vi "Two_tanks.vi"() -> ()   [LabVIEW 2016]
uses:
  <vilib>/Simulation/Scripting/Companion Diagram/SimConfigNode/SimParams.ctl
  <vilib>/Simulation/Scripting/Companion Diagram/SimConfigNode/_simSolvers.ctl
  <vilib>/Simulation/Implementation/Shared/SIMSCR Execution Mode.ctl
  <vilib>/Simulation/Param Hierarchy/Typedefs/SIMPH Param Control Actions.ctl
  <vilib>/Simulation/Implementation/Shared/SIM limit type.ctl
  <vilib>/Simulation/Implementation/Shared/NILVSim_ParamChanged.vi
  <vilib>/Simulation/Implementation/Shared/NILVSIM_BeginStep.vi
  <vilib>/Simulation/DataSources/Implementation/NILVSim Step.llb/SIM Step (scalar).vi
  <vilib>/Simulation/ContinuousLinear/Implementation/NILVSim Transfer Function.llb/SIM Transfer Function Distributor (SISO).vi
  <vilib>/Simulation/ContinuousLinear/Implementation/NILVSim Transfer Function.llb/SIM Transfer Function Collector (SISO).vi
  <vilib>/Simulation/ContinuousLinear/Implementation/NILVSim Integrator new.llb/SIM Integrator distributor (scalar).vi
  <vilib>/Simulation/SignalDisplay/Implementation/NILVSim Time Waveform.llb/SIM Time Waveform (vector).vi
  <vilib>/Simulation/ContinuousLinear/Implementation/NILVSim Integrator new.llb/SIM Integrator collector (scalar).vi
  <vilib>/Simulation/SignalDisplay/Implementation/NILVSim Time Waveform.llb/SIM Time Waveform (scalar).vi
  <vilib>/Simulation/Implementation/Shared/NILVSim_Manager.vi
  <vilib>/Utility/error.llb/Clear Errors.vi
  <vilib>/Simulation/Implementation/Shared/NILVSim_FinalizeModel.vi
  <vilib>/Simulation/Implementation/Shared/SIM Unbundle Sim Info.vi
  <vilib>/Simulation/Implementation/Shared/NILVSim_Initialize.vi
  <vilib>/Simulation/Utility/Implementation/NILVSim Get Time and IsAcceptedStep.vi
  <vilib>/Simulation/Implementation/Shared/SIMSH Read Queue.vi
  <vilib>/Simulation/Implementation/Shared/NILVSim_GetModelError.vi
  <vilib>/Simulation/Implementation/Shared/SIM Bundle Sim Info.vi
  <vilib>/Simulation/Scripting/Companion Diagram/SimConfigNode/SimDog.xnode
  <vilib>/Simulation/Implementation/XNodeFramework/SimXNode/SimX.xnode
  <vilib>/Simulation/ContinuousLinear/Implementation/NILVSim Integrator new.llb/SIM Integrator (scalar).vi
  <vilib>/Simulation/ContinuousLinear/Implementation/NILVSim Transfer Function.llb/SIM Transfer Function (SISO).vi
  <vilib>/Simulation/Implementation/Shared/NI_SIM_Implementation.lvlib
panel:
  in  "Transfer Function 4":cluster{"Numerator":dbl[], "Denominator":dbl[]}={"Numerator"=[3.68], "Denominator"=[1.0, 14.2]} {"Numerator" min=0.0 max=0.0; "Denominator" min=10.2 max=10.2}
  in  "h0(s) 3":dbl=0.5 min=4.0 max=4.0
  in  "Transfer Function 3":cluster{"Numerator":dbl[], "Denominator":dbl[]}={"Numerator"=[5.0], "Denominator"=[1.0, 13.15]} {"Denominator" min=10.2 max=10.2}
  in  "h0(s) 2":dbl=1.0 min=4.0 max=4.0
  out "F1 2":waveform(dbl)(graph)={"t0"=timestamp(50 s since 1904-01-01), "dt"=1.0, "Y"=[1.0971753787144658]}
  out "F2":dbl=2.096471574642852
  out "h2":dbl=1.09879826582137
  out "F1":dbl=1.0971753787144658
  out "h1":dbl=2.3025920774786015
  out "Depósito2":waveform(dbl)[](graph)=[{"t0"=timestamp(50 s since 1904-01-01), "dt"=1.0, "Y"=[1.0]}, {"t0"=timestamp(50 s since 1904-01-01), "dt"=1.0, "Y"=[1.09879826582137]}, {"t0"=timestamp(50 s since 1904-01-01), "dt"=1.0, "Y"=[2.2856012331833835]}]
  out "Deposito 2":dbl(slide)=1.09879826582137 scale=0.0..4.0
  in  "Deposito2: K1":dbl(slide)=2.0 scale=0.0..5.0
  in  "D2 q0":dbl=0.5
  in  "Deposito2: Area":dbl(slide)=2.0 scale=0.0..5.0
  in  "D2 h0":dbl=0.5
  in  "D2: q":dbl(slide)=0.5 scale=0.0..2.0
  in  "Deposito1: K1":dbl(slide)=1.0 scale=0.0..5.0
  in  "Deposito1: Area":dbl(slide)=3.0 scale=0.0..5.0
  in  "D1: q":dbl(slide)=0.1 scale=0.0..2.0
  out "Deposito 1":dbl(slide)=2.3025920774786015 scale=0.0..4.0
  out "Depósito1":waveform(dbl)[](graph)=[{"t0"=timestamp(50 s since 1904-01-01), "dt"=1.0, "Y"=[1.1]}, {"t0"=timestamp(50 s since 1904-01-01), "dt"=1.0, "Y"=[2.3025920774786015]}, {"t0"=timestamp(50 s since 1904-01-01), "dt"=1.0, "Y"=[1.4888409047912208]}]
  in  "D1 q0":dbl=1.0
  in  "D1 h0":dbl=1.0
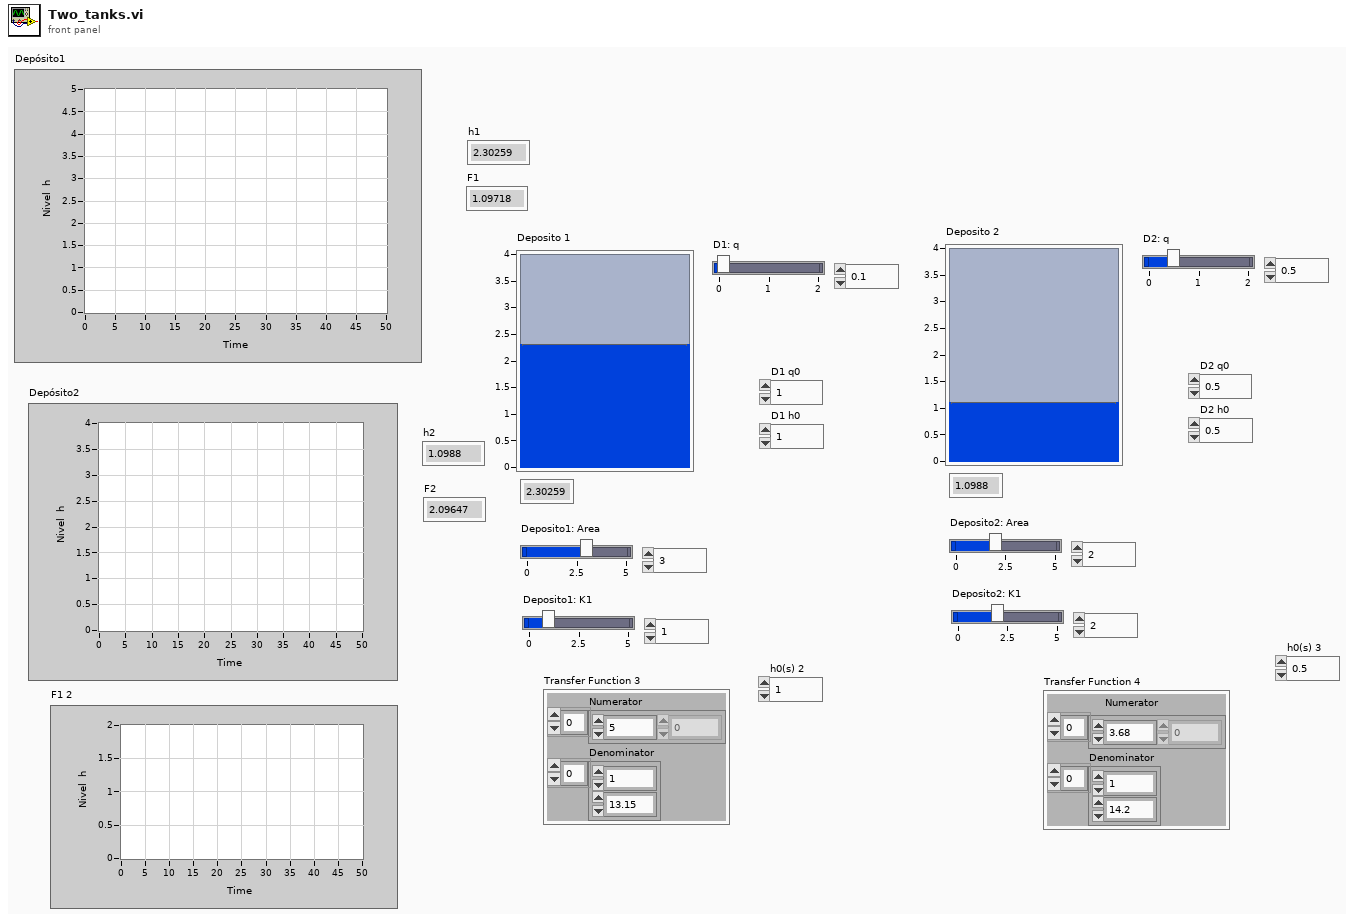
[diagram p1: front panel]
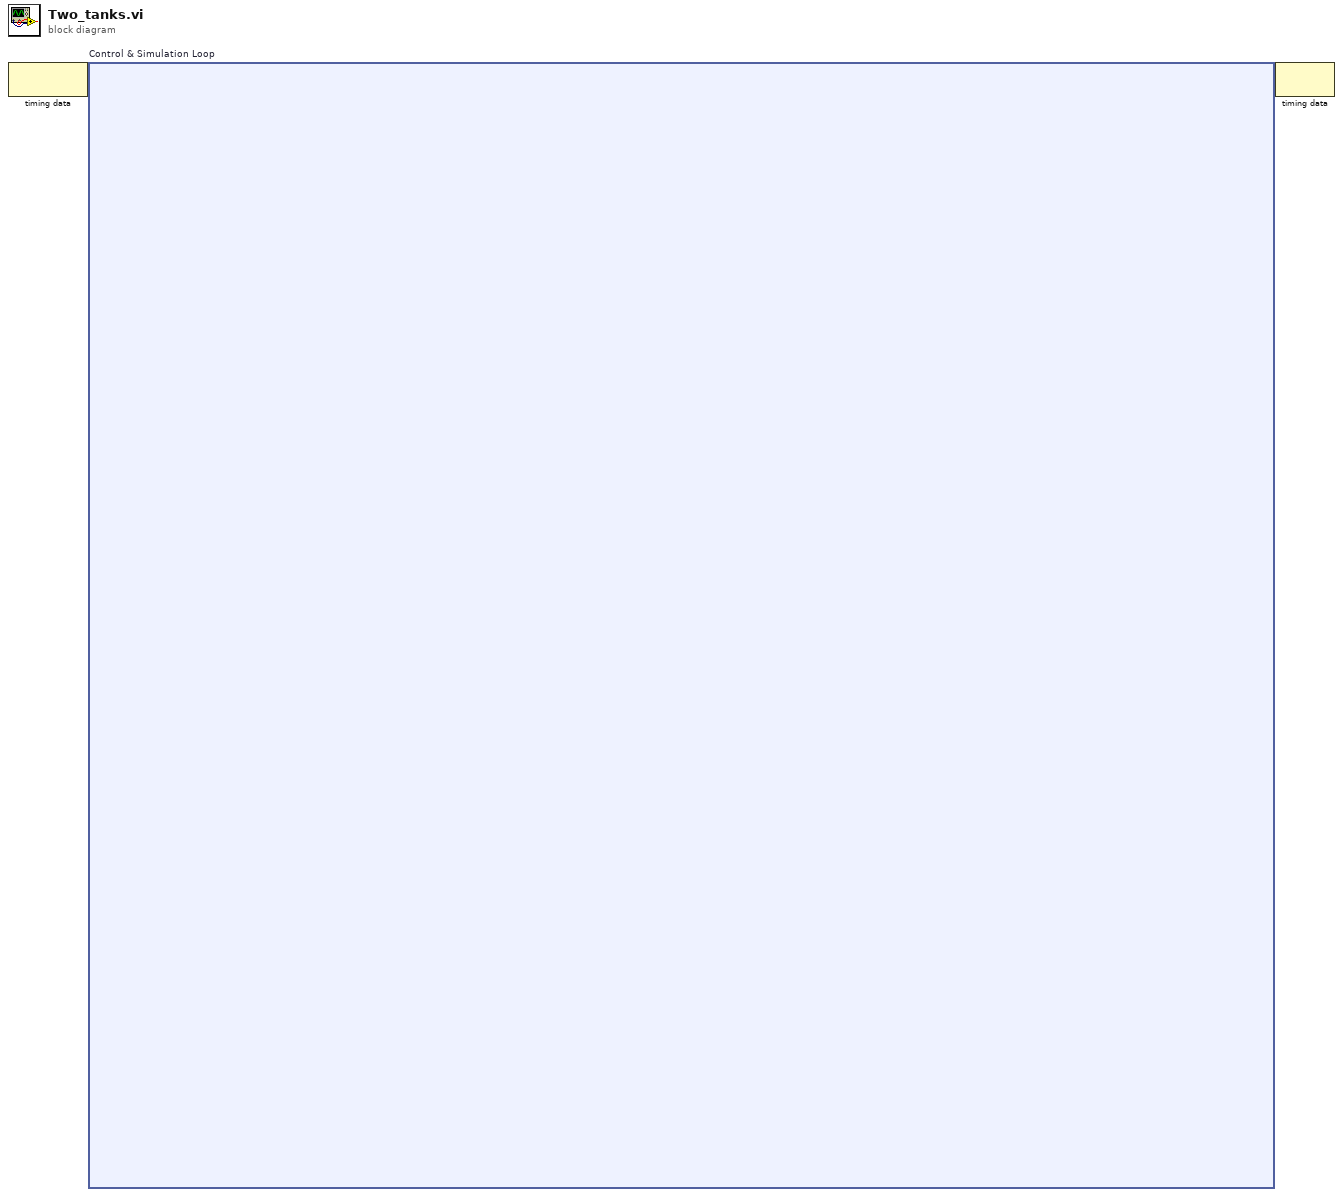
[diagram p0: block diagram]
diagram:
  n1 = node-c288() -> (w2:variant)  [unwired: 1 in]
  n2 = node-c254 "Control & Simulation Loop"(w2) -> (w1:variant)
  n3 = node-c288(w1) -> ()  [unwired: 1 out]
